vi "GetPersonnel.vi"(7 "LabVIEW Web Service Request":refnum<class "Web Request.lvclass">, 10 "Command":string, 11 "UID":string) -> (2 "Response":string)   [LabVIEW 2015]
uses:
  <vilib>/wsapi/Web Request.lvclass
  LVRestAPI/TypeDef/GetPersonnelCommands.ctl
  TypeDef/PersonnelActions.ctl
  LVRestAPI/PersonnelRestApi.lvlib
panel:
  out "postdata":string
  # "Use the Web Service Request input terminal to call the VIs on the Web Services palette. Do not remove it from the connector pane unless you don't need access to the palette."
  # "Each additional control wired to the connector pane will be available as an input in the URL. To include an indicator in terminal-mode output (the default setting), it must also be wired to the connector pane."
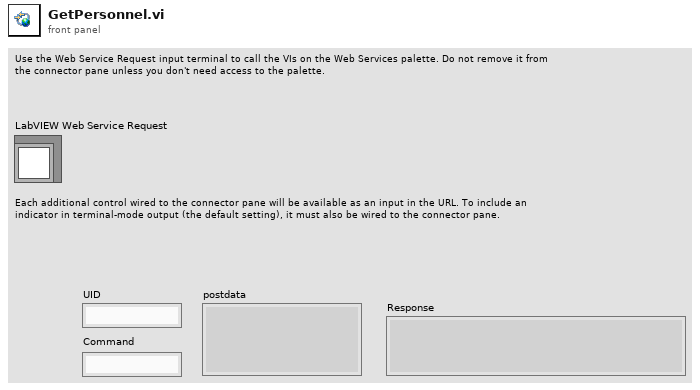
[diagram p1: front panel]
types:
  T1 = typedef "PersonnelRestApi.lvlib/GetPersonnelCommands.ctl" = enum16{"ReadPersonnel", "ReadName", "ReadRole", "ReadRequests", "ReadPUIDs"}
  T2 = typedef "PersonnelActions.ctl" = enum16{"Init", "Read Personnel", "Add Personnel", "Remove Personnel", "Read Name", "Write Name", "Read Role", "Write Role", "Read Requests", "Add Requests", "Remove Requests", "Read PUIDs"}
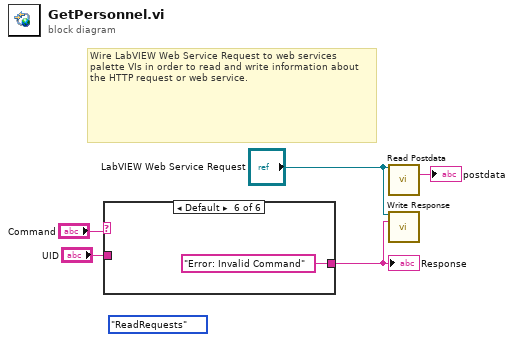
[diagram p0: block diagram]
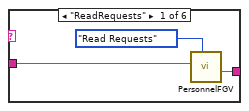
[diagram p2: hidden frame]
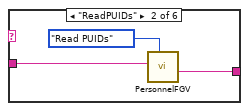
[diagram p3: hidden frame]
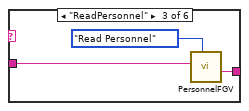
[diagram p4: hidden frame]
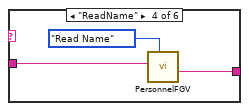
[diagram p5: hidden frame]
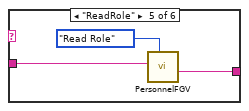
[diagram p6: hidden frame]
diagram:
  (unwired) GetPersonnelCommands."ReadRequests" ("Room Commands")
  # "Wire LabVIEW Web Service Request to web services palette VIs in order to read and write information about the HTTP request or web service."
  n1 = case shown="Default" "Command" {
    tunnel: "UID" -> [w8 w11 w14 w17 w20 _]
    tunnel: [w7 w10 w13 w16 w19 "Error: Invalid Command" ("Data Out")] -> w4
    frame "ReadRequests" {
      n2 = call "PersonnelFGV.vi"("Actions"=PersonnelActions."Read Requests", "PUID"=w8) -> ("Data Out"=w7:string)  [unwired: 8 in, 1 out]
    }
    frame "ReadPUIDs" {
      n3 = call "PersonnelFGV.vi"("Actions"=PersonnelActions."Read PUIDs", "PUID"=w11) -> ("Data Out"=w10:string)  [unwired: 8 in, 1 out]
    }
    frame "ReadPersonnel" {
      n4 = call "PersonnelFGV.vi"("Actions"=PersonnelActions."Read Personnel", "PUID"=w14) -> ("Data Out"=w13:string)  [unwired: 8 in, 1 out]
    }
    frame "ReadName" {
      n5 = call "PersonnelFGV.vi"("Actions"=PersonnelActions."Read Name", "PUID"=w17) -> ("Data Out"=w16:string)  [unwired: 8 in, 1 out]
    }
    frame "ReadRole" {
      n6 = call "PersonnelFGV.vi"("Actions"=PersonnelActions."Read Role", "PUID"=w20) -> ("Data Out"=w19:string)  [unwired: 8 in, 1 out]
    }
    frame Default {
    }
  }
  "Response" <- w4
  n7 = call <vilib>:"Read Postdata.vi"("LabVIEW Web Service Request"="LabVIEW Web Service Request") -> ("postdata"=→"postdata":string)  [unwired: 12 in, 2 out]
  n8 = call <vilib>:"Write Response.vi"("LabVIEW Web Service Request"="LabVIEW Web Service Request", "response string"=w4) -> ()  [unwired: 12 in, 2 out]
